vi "hydraharp_get_hardware_initialization_info.vi"(8 "error in (no error)":errorcluster, 11 "hydraharp in":refnum<class "hydraharp.lvclass">) -> (0 "error out":errorcluster, 2 "resulting string":string, 3 "hydraharp out":refnum<class "hydraharp.lvclass">)   [LabVIEW 2015, in "hydraharp.lvclass"]
uses:
  hydraharp.lvclass
  hydraharp.lvclass/hydraharp.ctl
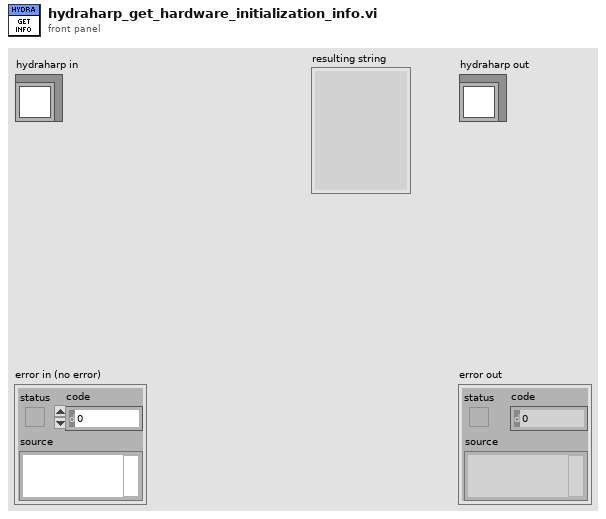
[diagram p1: front panel]
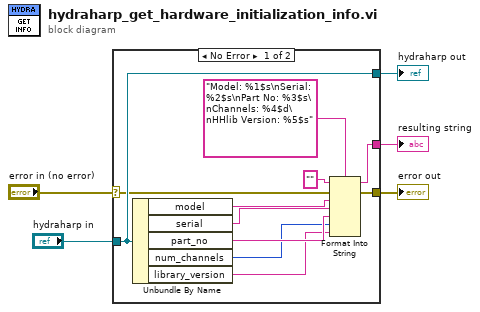
[diagram p0: block diagram]
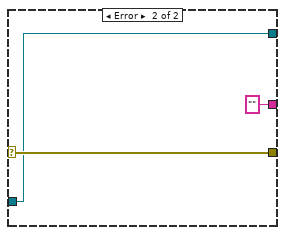
[diagram p2: hidden frame]
diagram:
  n1 = case shown="No Error" "error in (no error)" {
    selector: "error in (no error)" -> [w12 w19]
    tunnel: [w11 w19] -> w4
    tunnel: [w16 w18] -> w2
    tunnel: "hydraharp in" -> [w16 w18]
    tunnel: [w10 ""] -> w1
    frame No Error {
      n2 = Unbundle By Name(w16) -> ("model"=w14:string, "serial"=w9:string, "part_no"=w8:string, "num_channels"=w7:i32, "library_version"=w6:string)
      n3 = Format Into String(format string="Model: %1$s\nSerial: %2$s\nPart No: %3$s\nChannels: %4$d\nHHlib Version: %5$s", initial string="", error in=w12, w14, w9, w8, w7, w6) -> (resulting string=w10:string, error out=w11:errorcluster)
    }
    frame Error {
    }
  }
  "error out" <- w4
  "hydraharp out" <- w2
  "resulting string" <- w1
